vi "CS++DeviceBase-Content.vi"() -> (0 "CS++Classes & Messages":T1(array[cluster]))   [LabVIEW 2015]
doc: "Place actor and class constants that should be included included in an application on the blockdiagramm."
uses:
  <vilib>/ActorFramework/Message/Message.lvclass
  CS++DMM/CS++DMM.lvclass
  CS++DMMGui/CS++DMMGui.lvclass
  CS++DCPwr/CS++DCPwr.lvclass
  CS++DCPwrGui/CS++DCPwrGui.lvclass
  CS++Fgen/CS++Fgen.lvclass
  CS++FgenGui/CS++FgenGui.lvclass
  CS++Scope/CS++Scope.lvclass
  CS++ScopeGui/CS++ScopeGui.lvclass
  CS++MCS/CS++MCS.lvclass
  CS++Motor/CS++Motor.lvclass
  CS++MotorGui/CS++MotorGui.lvclass
  CSPP_Core/Actors/CS++BaseActor/CS++BaseActor.lvclass
panel:
  # "Place actor and class constants on the blockdiagramm."
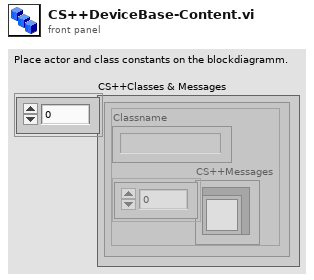
[diagram p1: front panel]
types:
  T1 = cluster{"Classname":string, "CS++Messages":refnum<class "Message.lvclass">[]}[]
  T2 = cluster{"class name":string, "CS++Messages":refnum<class "Message.lvclass">[]}
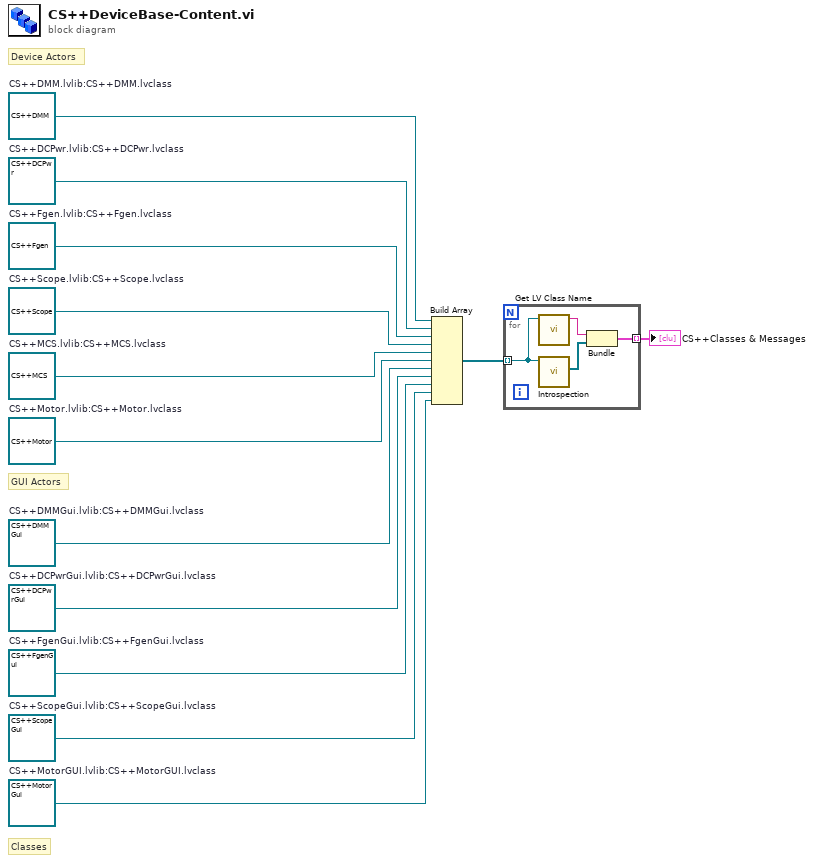
[diagram p0: block diagram]
diagram:
  w1 = refnum<class "CS++MotorGui.lvclass"> refnum  # CS++MotorGUI.lvlib:CS++MotorGUI.lvclass
  w2 = refnum<class "CS++Motor.lvclass"> refnum  # CS++Motor.lvlib:CS++Motor.lvclass
  w4 = refnum<class "CS++MCS.lvclass"> refnum  # CS++MCS.lvlib:CS++MCS.lvclass
  w5 = refnum<class "CS++ScopeGui.lvclass"> refnum  # CS++ScopeGui.lvlib:CS++ScopeGui.lvclass
  w10 = refnum<class "CS++Scope.lvclass"> refnum  # CS++Scope.lvlib:CS++Scope.lvclass
  w6 = refnum<class "CS++FgenGui.lvclass"> refnum  # CS++FgenGui.lvlib:CS++FgenGui.lvclass
  w11 = refnum<class "CS++Fgen.lvclass"> refnum  # CS++Fgen.lvlib:CS++Fgen.lvclass
  w7 = refnum<class "CS++DCPwrGui.lvclass"> refnum  # CS++DCPwrGui.lvlib:CS++DCPwrGui.lvclass
  w12 = refnum<class "CS++DCPwr.lvclass"> refnum  # CS++DCPwr.lvlib:CS++DCPwr.lvclass
  w3 = refnum<class "CS++DMMGui.lvclass"> refnum  # CS++DMMGui.lvlib:CS++DMMGui.lvclass
  w13 = refnum<class "CS++DMM.lvclass"> refnum  # CS++DMM.lvlib:CS++DMM.lvclass
  # "Classes"
  # "GUI Actors"
  # "Device Actors"
  n1 = Build Array(w13, w12, w11, w10, w4, w2, w3, w7, w6, w5, w1) -> (w8:refnum<class "CS++BaseActor.lvclass">[])
  n2 = for {
    tunnel: w8 -> [w17] mode=indexing
    tunnel: [w14] -> w9 mode=indexing
    n3 = call <vilib>:"Get LV Class Name.vi"("object"=w17) -> ("class name"=w16:string)  [unwired: 9 in, 1 out]
    n4 = call "Introspection.vi"("CS++BaseActor in"=w17) -> ("CS++Messages"=w15:refnum<class "Message.lvclass">[])  [unwired: 8 in, 2 out]
    n5 = Bundle("class name"=w16, "CS++Messages"=w15) -> (w14:T2)  [unwired: 1 in]
  }
  "CS++Classes & Messages" <- w9
